vi "AlliGator Ordered Available Channel Names.vi"(8 "error in (no error)":errorcluster, 11 "Channel Names":string[](array[string])) -> (0 "error out":errorcluster, 3 "Ordered Channel Names":string[](array[string]))   [LabVIEW 2021, in "AlliGator Files.lvlib"]
doc: "Reorders channel names to put that corresponding to G2 first."
uses:
  AlliGator Files.lvlib
panel:
  # "see the AlliGator License on the block diagram (Ctrl+E or Window:Show Block Diagram)"
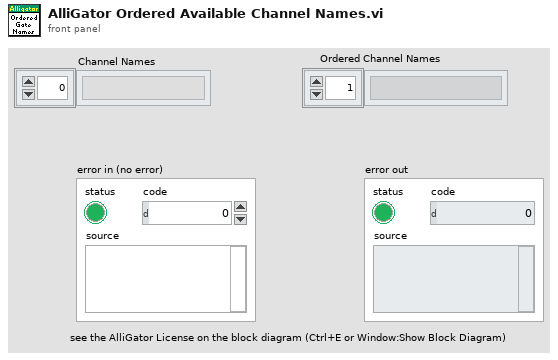
[diagram p1: front panel]
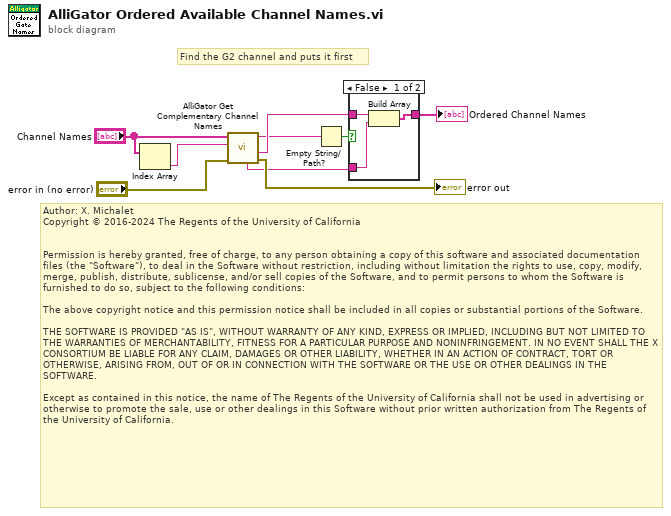
[diagram p0: block diagram]
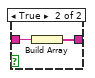
[diagram p2: hidden frame]
diagram:
  # "Author: X. Michalet\nCopyright © 2016-2024 The Regents of the University of California\n \n\nPermission is hereby granted, free of charge, to any person obtaining a copy of this software and associated documentation files (the \"Software\"), to deal in the Software without restriction, including without limitation the rights to use, copy, modify, merge, publish, distribute, sublicense, and/or sell copies of the Software, and to permit persons to whom the Software is furnished to do so, subject to the following conditions:\n\nThe above copyright notice and this permission notice shall be included in all copies or substantial portions of the Software.\n\nTHE SOFTWARE IS PROVIDED \"AS IS\", WITHOUT WARRANTY OF ANY KIND, EXPRESS OR IMPLIED, INCLUDING BUT NOT LIMITED TO THE WARRANTIES OF MERCHANTABILITY, FITNESS FOR A PARTICULAR PURPOSE AND NONINFRINGEMENT. IN NO EVENT SHALL THE X CONSORTIUM BE LIABLE FOR ANY CLAIM, DAMAGES OR OTHER LIABILITY, WHETHER IN AN ACTION OF CONTRACT, TORT OR OTHERWISE, ARISING FROM, OUT OF OR IN CONNECTION WITH THE SOFTWARE OR THE USE OR OTHER DEALINGS IN THE SOFTWARE.\n\nExcept as contained in this notice, the name of The Regents of the University of California shall not be used in advertising or otherwise to promote the sale, use or other dealings in this Software without prior written authorization from The Regents of the University of California."
  # "Find the G2 channel and puts it first"
  n1 = Index Array(array="Channel Names") -> (element=w4:string)  [unwired: 1 in]
  n2 = call "AlliGator Get Complementary Channel Names.vi"("Error In"="error in (no error)", "Selected Channel Name"=w4, "Available Channel Names"="Channel Names") -> ("Error Out"=→"error out":errorcluster, "G2 Channel Name (or single Gate Name)"=w8:string, "Complementary Channel Name (or empty)"=w2:string, "INT Channel Name (or empty)"=w1:string)  [unwired: 3 in, 2 out]
  n3 = Empty String/Path?(string/path=w2) -> (empty?=w7:bool)
  n4 = case shown="False" w7 {
    tunnel: w8 -> [w12 w14]
    tunnel: [w11 w13] -> w9
    tunnel: w1 -> [w10 _]
    frame False {
      n5 = Build Array(w12, w10) -> (w11:string[])
    }
    frame True {
      n6 = Build Array(w14) -> (w13:string[])
    }
  }
  "Ordered Channel Names" <- w9
